vi "Autonomous Independent.vi"() -> ()   [LabVIEW 2011]
doc: "This VI is called when autonomous begins, and will automatically be terminated when autonomous ends. You can carry out timed or sensor driven robot movement independently without needing to return to the caller."
uses:
  <vilib>/Rock Robotics/WPI/Relay/WPI_RelayValue.ctl
  Robot Global Data.vi
  cupStateGlobal.vi
  <vilib>/Rock Robotics/WPI/RobotDrive/WPI_RobotDriveArcadeDrive_Standard(NoSaturation).vi
panel:
  out "Fixed Distance[m]":dbl
  in  "MotorPower 3":dbl
  in  "Slide 3":dbl(slide) scale=400.0..2000.0
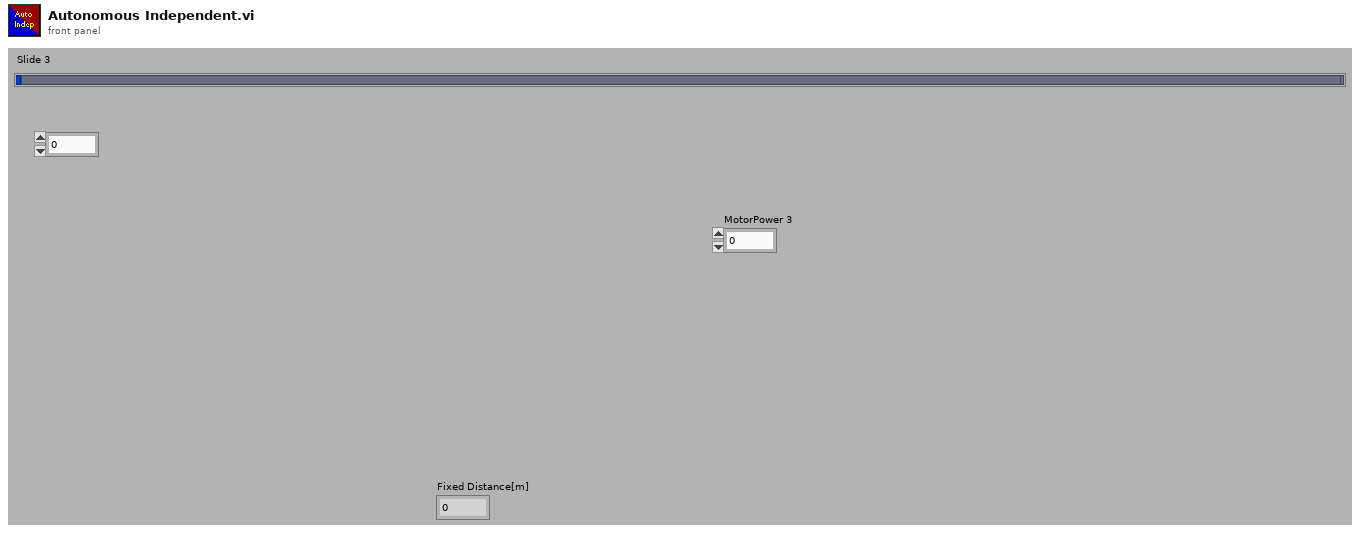
[diagram p1: front panel]
types:
  T1 = typedef "WPI_JoystickDevRef.ctl" = cluster{"Device":T2}
  T2 = typedef "WPI_JoystickDeviceEnum.ctl" = enum16{"USB 1", "USB 2", "USB 3", "USB 4", "Kinect 1", "Kinect 2"}
  T3 = typedef "WPI_DigitalInputDevRef.ctl" = cluster{"DevStatus":errorcluster, "DIO Channel":T4, "Digital Module":T5}
  T4 = typedef "FPGA_DIOChannel.ctl" = enum8{"DIO 1", "DIO 2", "DIO 3", "DIO 4", "DIO 5", "DIO 6", "DIO 7", "DIO 8", "DIO 9", "DIO 10", "DIO 11", "DIO 12", "DIO 13", "DIO 14", "Invalid"}
  T5 = typedef "FPGA_TypedefDigitalModule.ctl" = enum16{"Digital Module 1", "Digital Module 2"}
  T6 = typedef "WPI_RelayValue.ctl" = enum16{"Off", "On", "Forward", "Reverse"}
  T7 = typedef "WPI_RobotDriveDevRef.ctl" = cluster{"DevStatus":errorcluster, "Motors[]":T8[], "Square Inputs":bool, "Max Output":dbl, "Isochronous":bool}
  T8 = typedef "WPI_MotorControlDeviceRef.ctl" = cluster{"DeviceStatus":errorcluster, "Type":enum16{"PWM", "CAN"}, "PWM":cluster{"Digital Module":T5, "PWM Channel":T9, "DeadBand":T10}, "CAN":cluster{"Device Number":u8, "Control Mode":T11, "Semaphore":T12, "Max Vout":dbl}, "Invert":bool, "TransformRef":T13, "InvTransformRef":T13}
  T9 = typedef "FPGA_DIOPWMChannel.ctl" = enum8{"PWM 1", "PWM 2", "PWM 3", "PWM 4", "PWM 5", "PWM 6", "PWM 7", "PWM 8", "PWM 9", "PWM 10", "Invalid"}
  T10 = typedef "WPI_PWMDeadband.ctl" = cluster{"Name":string, "maxPositivePwm":i32, "minPositivePwm":i32, "centerPwm":i32, "maxNegativePwm":i32, "minNegativePwm":i32, "angularRange":u16}
  T11 = typedef "WPI_CANJaguar_ControlMode.ctl" = enum8{"Percent VBus", "Current", "Speed", "Position", "Voltage"}
  T12 = typedef "Semaphore RefNum" = refnum<k1>
  T13 = typedef "WPI_PWMTransform_ConPane.ctl" = refnum<vi>
  T14 = typedef "WPI_EncoderDevRef.ctl" = cluster{"DevStatus":errorcluster, "EncoderIndex":T15, "CounterIndex":T16, "DistancePerCount":dbl, "Decoding Type":T17}
  T15 = typedef "FPGA_EncoderIdx.ctl" = enum8{"Enc 0", "Enc 1", "Enc 2", "Enc 3", "Invalid"}
  T16 = typedef "FPGA_CounterCtrSystemIndex.ctl" = enum8{"Ctr 0", "Ctr 1", "Ctr 2", "Ctr 3", "Ctr 4", "Ctr 5", "Ctr 6", "Ctr 7", "Invalid"}
  T17 = typedef "WPI_EncoderType.ctl" = enum16{"1x", "2x", "4x"}
  T18 = typedef "WPI_AnalogChannelDevRef.ctl" = cluster{"DevStatus":errorcluster, "Analog Module":T19, "Analog Channel":T20}
  T19 = typedef "FPGA_TypedefAnalogModule.ctl" = enum16{"Analog Module 1", "Analog Module 2"}
  T20 = typedef "FPGA_AIChannel.ctl" = enum8{"AI 1", "AI 2", "AI 3", "AI 4", "AI 5", "AI 6", "AI 7", "AI 8", "Invalid"}
  T21 = cluster{"RightAxis":dbl, "LeftAxis":dbl, "RightHead":bool, "Left Head":bool, "Left Leg Out":bool, "Left Leg Forward":bool, "Left Leg Back":bool, "Right Leg Out":bool, "Right Leg Forward":bool, "Right Leg Back":bool}
  T22 = typedef "WPI_RelayDevRef.ctl" = cluster{"DevStatus":errorcluster, "Relay Channel":T23, "Digital Module":T5, "Relay Direction":T24}
  T23 = typedef "FPGA_DIORelayChannel.ctl" = enum8{"Relay 1", "Relay 2", "Relay 3", "Relay 4", "Relay 5", "Relay 6", "Relay 7", "Relay 8", "Invalid"}
  T24 = typedef "WPI_RelayDirection.ctl" = enum16{"Both directions", "Forward only", "Reverse only"}
  T25 = typedef "WPI_ServoDeviceRef.ctl" = cluster{"DeviceStatus":errorcluster, "Digital Module":T5, "PWM Channel":T9, "DeadBand":T10}
  T26 = cluster{"Position":cluster{"X":dbl, "Y":dbl}, "Distance (m)":dbl, "Target Found?":bool}
  T27 = cluster{"axis 1 (x)":dbl, "axis 2 (y)":dbl, "axis 3 (throttle)":dbl, "axis 4":dbl, "axis 5":dbl, "axis 6":dbl}
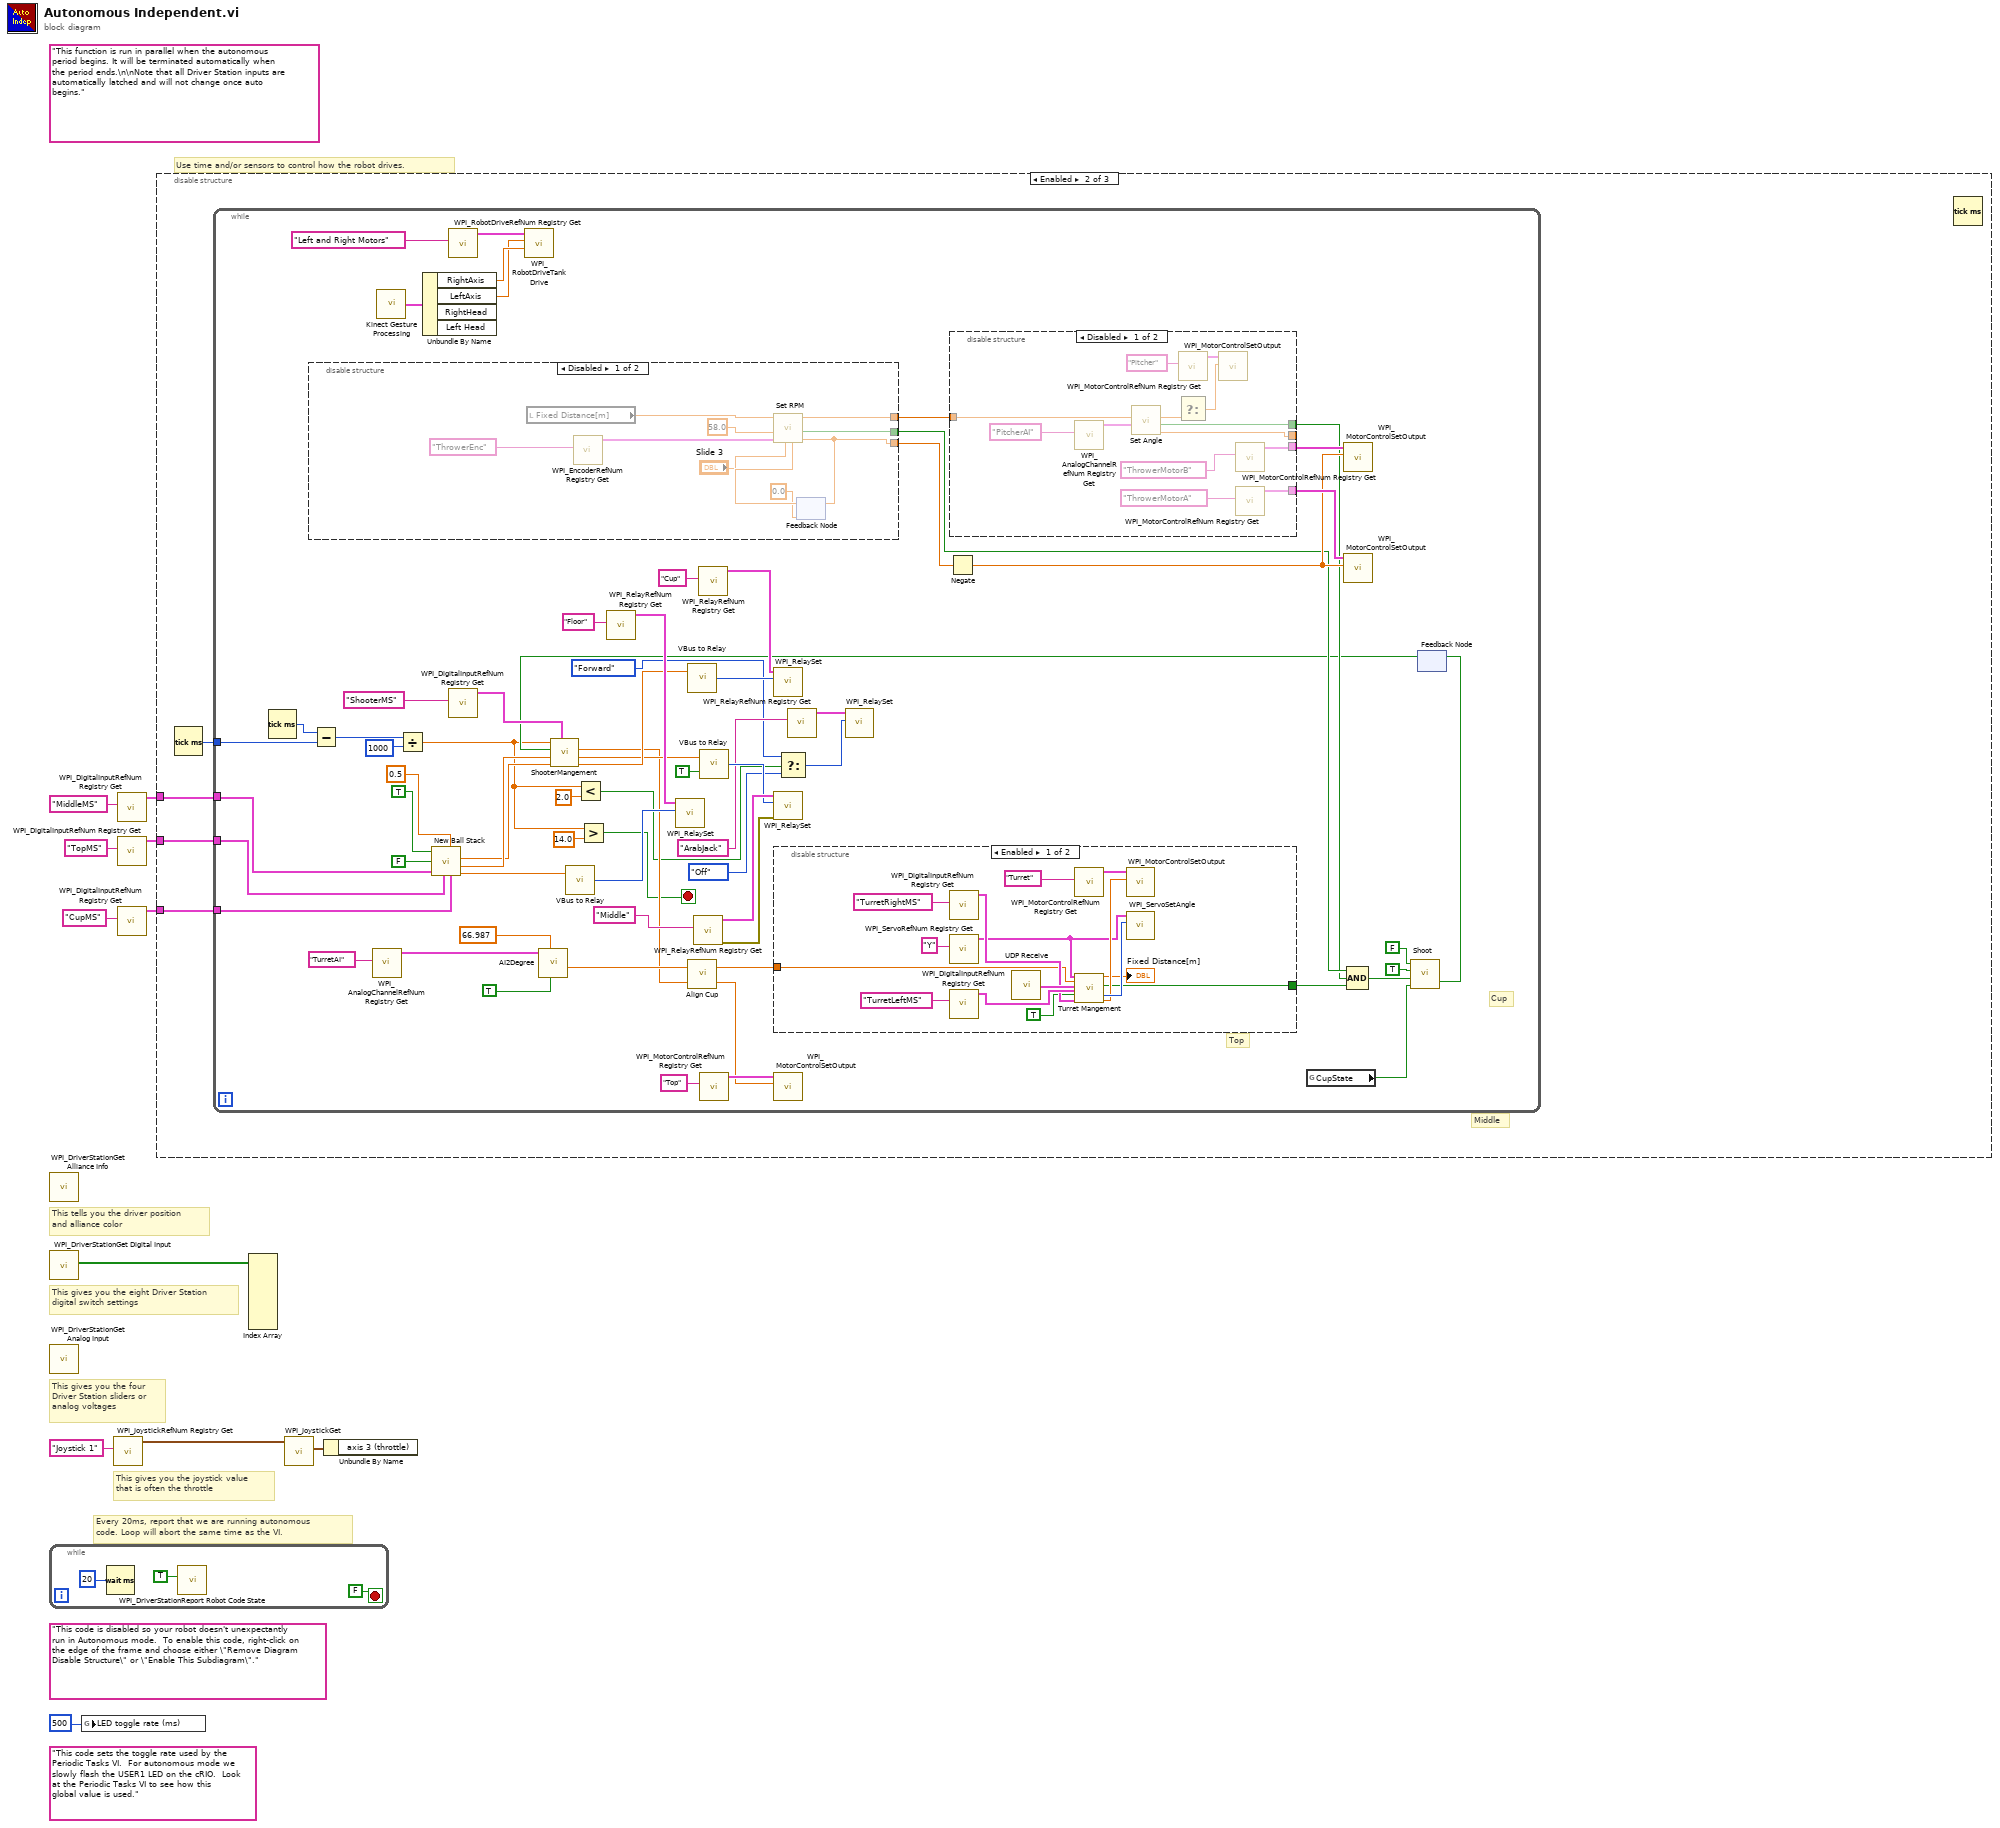
[diagram p0: block diagram]
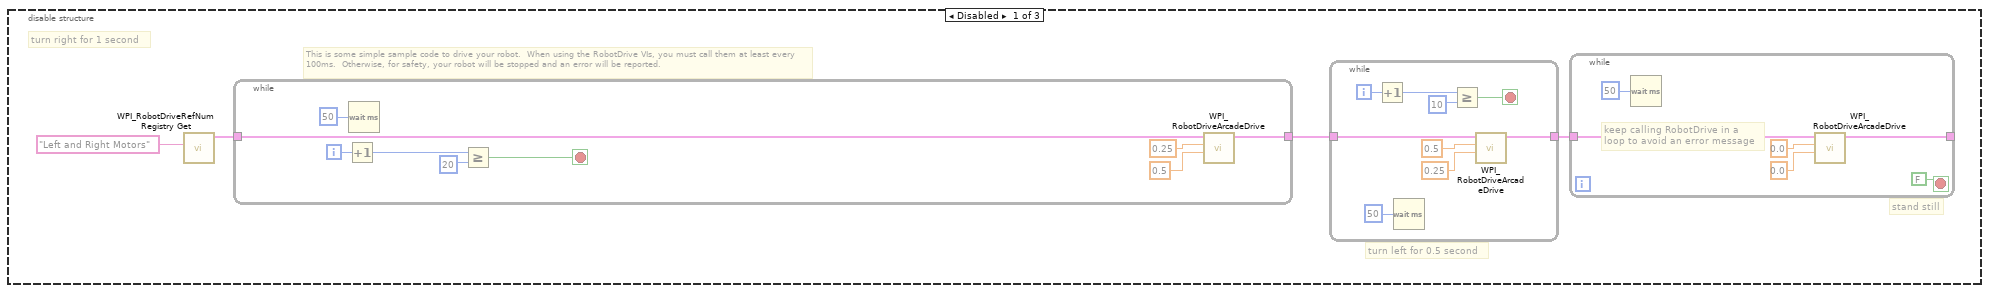
[diagram p2: hidden frame]
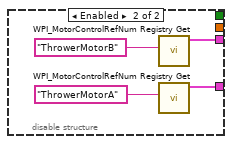
[diagram p4: hidden frame]
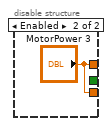
[diagram p5: hidden frame]
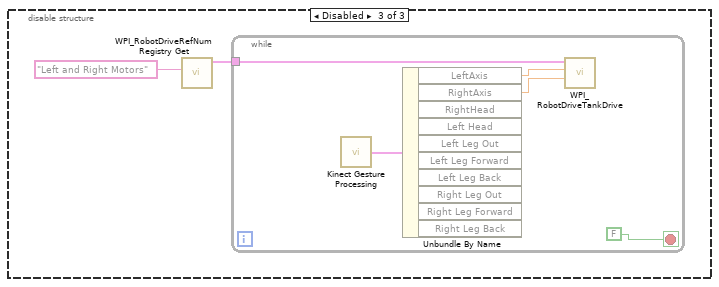
[diagram p6: hidden frame]
diagram:
  (unwired) "This code sets the toggle rate used by the Periodic Tasks VI.  For autonomous mode we slowly flash the USER1 LED on the cRIO.  Look at the Periodic Tasks VI to see how this global value is used."
  (unwired) "This code is disabled so your robot doesn't unexpectantly run in Autonomous mode.  To enable this code, right-click on the edge of the frame and choose either \"Remove Diagram Disable Structure\" or \"Enable This Subdiagram\"."
  (unwired) "This function is run in parallel when the autonomous period begins. It will be terminated automatically when the period ends.\n\nNote that all Driver Station inputs are automatically latched and will not change once auto begins."
  # "Every 20ms, report that we are running autonomous\ncode. Loop will abort the same time as the VI."
  # "This gives you the joystick value\nthat is often the throttle"
  # "Use time and/or sensors to control how the robot drives."
  # "This tells you the driver position\nand alliance color"
  # "This gives you the eight Driver Station\ndigital switch settings"
  # "This gives you the four\nDriver Station sliders or\nanalog voltages"
  n1 = call <vilib>:"WPI_DriverStationGet Alliance Info.vi"() -> ()  [unwired: 12 out]
  n2 = call <vilib>:"WPI_DriverStationGet Digital Input.vi"() -> ("Driver Station Digital Input (1-8)"=w11:bool[])  [unwired: 11 out]
  n3 = call <vilib>:"WPI_DriverStationGet Analog Input.vi"() -> ()  [unwired: 12 out]
  n4 = while {
    stop <- FALSE stop-if-true
    n5 = Wait (ms)(milliseconds to wait=u32 20) -> ()  [unwired: 1 out]
    n6 = call <vilib>:"WPI_DriverStationReport Robot Code State.vi"("Autonomous"=TRUE) -> ()  [unwired: 10 in, 1 out]
  }
  n7 = global write "Robot Global Data.vi" "LED toggle rate (ms)"(u32 500 ("LED ms toggle rate")) -> ()
  n8 = call <vilib>:"WPI_JoystickRefNum Registry Get.vi"("refnum name"="Joystick 1") -> ("JoystickDevRef"=w8:T1)  [unwired: 1 in, 9 out]
  n9 = call <vilib>:"WPI_DigitalInputRefNum Registry Get.vi"("refnum name"="MiddleMS") -> ("DigitalInputDevRef"=w1:T3)  [unwired: 9 in, 1 out]
  n10 = call <vilib>:"WPI_DigitalInputRefNum Registry Get.vi"("refnum name"="TopMS") -> ("DigitalInputDevRef"=w2:T3)  [unwired: 9 in, 1 out]
  n11 = call <vilib>:"WPI_DigitalInputRefNum Registry Get.vi"("refnum name"="CupMS") -> ("DigitalInputDevRef"=w3:T3)  [unwired: 9 in, 1 out]
  n12 = disable-structure shown="Enabled" {
    disable-tunnel: w3 -> [_ w45 _]
    disable-tunnel: w2 -> [_ w46 _]
    disable-tunnel: w1 -> [_ w44 _]
    frame Disabled {
      # "This is some simple sample code to drive your robot.  When using the RobotDrive VIs, you must call them at least every 100ms.  Otherwise, for safety, your robot will be stopped and an error will be reported."
      # "stand still"
      # "turn left for 0.5 second"
      # "turn right for 1 second"
      n13 = call <vilib>:"WPI_RobotDriveRefNum Registry Get.vi"("refnum name"="Left and Right Motors") -> ("RobotDriveDevRef"=w17:T7)  [unwired: 1 in, 9 out]
      n14 = while {
        tunnel: w17 -> [w42]
        tunnel: [w35] -> w16
        i -> [w38]
        stop <- w36 stop-if-true
        n15 = Increment(x=w38) -> (x+1=w34:i32)
        n16 = Wait (ms)(milliseconds to wait=u32 50) -> ()  [unwired: 1 out]
        n17 = Greater Or Equal?(x=w34, y=20) -> (x >= y?=w36:bool)
        n18 = call-poly <vilib>:"WPI_RobotDriveArcadeDrive.vi"("Y axis value"=0.5 ("X axis value"), "X axis value"=0.25, "RobotDriveDevRef"=w42) -> ("RobotDriveDevRef"=w35:T7)  [unwired: 1 in, 7 out]
      }
      n19 = while {
        tunnel: w16 -> [w33]
        tunnel: [w26] -> w15
        i -> [w29]
        stop <- w27 stop-if-true
        n20 = Increment(x=w29) -> (x+1=w25:i32)
        n21 = Wait (ms)(milliseconds to wait=u32 50) -> ()  [unwired: 1 out]
        n22 = Greater Or Equal?(x=w25, y=10) -> (x >= y?=w27:bool)
        n23 = call-poly <vilib>:"WPI_RobotDriveArcadeDrive.vi"("Y axis value"=0.25 ("X axis value"), "X axis value"=0.5, "RobotDriveDevRef"=w33) -> ("RobotDriveDevRef"=w26:T7)  [unwired: 1 in, 7 out]
      }
      n24 = while {
        tunnel: w15 -> [w24]
        tunnel: [w20] -> _
        stop <- FALSE stop-if-true
        # "keep calling RobotDrive in a loop to avoid an error message"
        n25 = Wait (ms)(milliseconds to wait=u32 50) -> ()  [unwired: 1 out]
        n26 = call-poly <vilib>:"WPI_RobotDriveArcadeDrive.vi"("Y axis value"=0.0 ("X axis value"), "X axis value"=0.0, "RobotDriveDevRef"=w24) -> ("RobotDriveDevRef"=w20:T7)  [unwired: 1 in, 7 out]
      }
    }
    frame Enabled {
      # "Middle"
      n27 = Tick Count (ms)() -> (millisecond timer value=w43:u32)
      n28 = while {
        tunnel: w46 -> [w102]
        tunnel: w45 -> [w101]
        tunnel: w44 -> [w100]
        tunnel: w43 -> [w63]
        stop <- w60 stop-if-true
        # "Top"
        # "Cup"
        n29 = Tick Count (ms)() -> (millisecond timer value=w62:u32)
        n30 = disable-structure shown="Disabled" {
          disable-tunnel: [w155 _] -> w74
          disable-tunnel: [w150 "MotorPower 3"] -> w109
          disable-tunnel: [w149 "MotorPower 3"] -> w106
          frame Disabled {
            n31 = local read "Fixed Distance[m]"() -> (w146:dbl)
            n32 = call <vilib>:"WPI_EncoderRefNum Registry Get.vi"("refnum name"="ThrowerEnc") -> ("EncoderDevRef"=w154:T14)  [unwired: 9 in, 1 out]
            n33 = feedback #1(0.0 ("Thrower Voltage")) -> (w152:dbl)
            n34 = call "Set RPM.vi"("Last Thrower Voltage (node)"=w152, "Position"="Slide 3", "EncoderDevRef"=w154, "Angle"=58.0, "horizontal distance to basket"=w146) -> ("Thrower Voltage"=w149:dbl, "RPM SET"=w155:bool, "angle"=w150:dbl)  [unwired: 4 in]
            n35 = feedback-in #1(w149) -> ()
          }
          frame Enabled {
          }
        }
        n36 = Subtract(x=w62, y=w63) -> (x-y=w64:u32)
        n37 = call <vilib>:"WPI_AnalogChannelRefNum Registry Get.vi"("refnum name"="TurretAI") -> ("AIDeviceRef"=w84:T18)  [unwired: 9 in, 1 out]
        n38 = call "Kinect Gesture Processing.vi"() -> ("Joystick Data"=w51:T21)  [unwired: 1 in]
        n39 = Divide(x=w64, y=u32 1000 ("milliseconds to wait")) -> (x/y=w57:dbl)
        n40 = Unbundle By Name(w51) -> ("RightAxis"=w50:dbl, "LeftAxis"=w49:dbl)  [unwired: 2 out]
        n41 = call "New Ball Stack.vi"("Suck?"=TRUE, "spinOut?"=FALSE, "MiddleMS"=w100, "TopMS"=w102, "Top Stack Speed"=0.5, "CupMS"=w101) -> ("Top"=w98:dbl, "Middle"=w99:dbl, "Floor"=w77:dbl)  [unwired: 2 in]
        n42 = call <vilib>:"WPI_RobotDriveRefNum Registry Get.vi"("refnum name"="Left and Right Motors") -> ("RobotDriveDevRef"=w48:T7)  [unwired: 9 in, 1 out]
        n43 = call <vilib>:"WPI_DigitalInputRefNum Registry Get.vi"("refnum name"="ShooterMS") -> ("DigitalInputDevRef"=w96:T3)  [unwired: 9 in, 1 out]
        n44 = call <vilib>:"WPI_RobotDriveTankDrive.vi"("Right axis value"=w50, "Left axis value"=w49, "RobotDriveDevRef"=w48) -> ()  [unwired: 7 in, 2 out]
        n45 = call "AI2Degree.vi"("Invert"=TRUE, "Calibrate"=66.987 ("y"), "AIDeviceRef"=w84) -> ("Degree"=w82:dbl)  [unwired: 8 in]
        n46 = call "VBus to Relay.vi"("Motor VBus"=w77) -> ("RelayValue"=w81:T6)  [unwired: 1 in]
        n47 = Less?(x=w57, y=2.0) -> (x < y?=w55:bool)
        n48 = Greater?(x=w57, y=14.0) -> (0:w60:bool)
        n49 = call <vilib>:"WPI_RelayRefNum Registry Get.vi"("refnum name"="Floor") -> ("RelayDevRef"=w110:T22)  [unwired: 9 in, 1 out]
        n50 = call <vilib>:"WPI_RelaySet.vi"("RelayValue"=w81, "RelayDevRef"=w110) -> ()  [unwired: 8 in, 2 out]
        n51 = call <vilib>:"WPI_RelayRefNum Registry Get.vi"("refnum name"="Middle") -> ("error out"=w91:errorcluster, "RelayDevRef"=w92:T22)  [unwired: 9 in]
        n52 = call <vilib>:"WPI_RelayRefNum Registry Get.vi"("refnum name"="Cup") -> ("RelayDevRef"=w112:T22)  [unwired: 9 in, 1 out]
        n53 = call <vilib>:"WPI_MotorControlRefNum Registry Get.vi"("refnum name"="Top") -> ("MotorControlDevRef"=w87:T8)  [unwired: 9 in, 1 out]
        n54 = Select(t=WPI_RelayValue."Forward" ("RelayValue"), s=w55, f=WPI_RelayValue."Off" ("RelayValue")) -> (s? t:f=w52:T6)
        n55 = call <vilib>:"WPI_RelayRefNum Registry Get.vi"("refnum name"="ArabJack") -> ("RelayDevRef"=w59:T22)  [unwired: 9 in, 1 out]
        n56 = call <vilib>:"WPI_RelaySet.vi"("RelayValue"=w52, "RelayDevRef"=w59) -> ()  [unwired: 8 in, 2 out]
        n57 = Negate(x=w106) -> (-x=w75:dbl)
        n58 = disable-structure shown="Disabled" {
          disable-tunnel: [w141 _] -> w73
          disable-tunnel: w109 -> [w129 _]
          disable-tunnel: [w138 w143] -> w108
          disable-tunnel: [w137 w142] -> w107
          disable-tunnel: [w132 _] -> _
          frame Disabled {
            n59 = call <vilib>:"WPI_AnalogChannelRefNum Registry Get.vi"("refnum name"="PitcherAI") -> ("AIDeviceRef"=w134:T18)  [unwired: 9 in, 1 out]
            n60 = call "Set Angle.vi"("AIDeviceRef"=w134, "Angle"=w129) -> ("Current Angle(above Horizon)"=w132:dbl, "Angle SET"=w141:bool, "Angle Motor"=w130:dbl)  [unwired: 7 in]
            n61 = call <vilib>:"WPI_MotorControlRefNum Registry Get.vi"("refnum name"="Pitcher") -> ("MotorControlDevRef"=w133:T8)  [unwired: 9 in, 1 out]
            n62 = Select(f=w130) -> (s? t:f=w131:dbl)  [unwired: 2 in]
            n63 = call <vilib>:"WPI_MotorControlSetOutput.vi"("Output"=w131, "MotorControlDevRef"=w133) -> ()  [unwired: 8 in, 2 out]
            n64 = call <vilib>:"WPI_MotorControlRefNum Registry Get.vi"("refnum name"="ThrowerMotorB") -> ("MotorControlDevRef"=w137:T8)  [unwired: 9 in, 1 out]
            n65 = call <vilib>:"WPI_MotorControlRefNum Registry Get.vi"("refnum name"="ThrowerMotorA") -> ("MotorControlDevRef"=w138:T8)  [unwired: 9 in, 1 out]
          }
          frame Enabled {
            n66 = call <vilib>:"WPI_MotorControlRefNum Registry Get.vi"("refnum name"="ThrowerMotorB") -> ("MotorControlDevRef"=w142:T8)  [unwired: 9 in, 1 out]
            n67 = call <vilib>:"WPI_MotorControlRefNum Registry Get.vi"("refnum name"="ThrowerMotorA") -> ("MotorControlDevRef"=w143:T8)  [unwired: 9 in, 1 out]
          }
        }
        n68 = global read "cupStateGlobal.vi" "CupState"() -> (w68:bool)
        n69 = call <vilib>:"WPI_MotorControlSetOutput.vi"("Output"=w75, "MotorControlDevRef"=w107) -> ()  [unwired: 8 in, 2 out]
        n70 = call <vilib>:"WPI_MotorControlSetOutput.vi"("Output"=w75, "MotorControlDevRef"=w108) -> ()  [unwired: 8 in, 2 out]
        n71 = feedback #2() -> (w66:bool)  [unwired: 1 in]
        n72 = call "ShooterMangement.vi"("Shooter MS"=w96, "Top"=w98, "Middle"=w99, "Le Shoot"=w66, "TeleOp Elapsed Seconds"=w57) -> ("Cup Gain"=w95:dbl, "Middle"=w88:dbl, "Top"=w78:dbl)  [unwired: 4 in]
        n73 = call "VBus to Relay.vi"("Motor VBus"=w95) -> ("RelayValue"=w94:T6)  [unwired: 1 in]
        n74 = call "Align Cup.vi"("Top Input"=w78, "Turret Angle"=w82) -> ("Top Output"=w80:dbl, "Turret Output"=w76:dbl)
        n75 = call "VBus to Relay.vi"("Invert Relay? (F)"=TRUE, "Motor VBus"=w88) -> ("RelayValue"=w89:T6)
        n76 = call <vilib>:"WPI_RelaySet.vi"("RelayValue"=w94, "RelayDevRef"=w112) -> ()  [unwired: 8 in, 2 out]
        n77 = call <vilib>:"WPI_RelaySet.vi"("error in (no error)"=w91, "RelayValue"=w89, "RelayDevRef"=w92) -> ()  [unwired: 7 in, 2 out]
        n78 = disable-structure shown="Enabled" {
          disable-tunnel: w76 -> [w116 _]
          disable-tunnel: [w115 _] -> w72
          frame Enabled {
            n79 = call <vilib>:"WPI_DigitalInputRefNum Registry Get.vi"("refnum name"="TurretRightMS") -> ("DigitalInputDevRef"=w120:T3)  [unwired: 9 in, 1 out]
            n80 = call <vilib>:"WPI_ServoRefNum Registry Get.vi"("refnum name"="Y") -> ("ServoDeviceRef"=w117:T25)  [unwired: 9 in, 1 out]
            n81 = call <vilib>:"WPI_DigitalInputRefNum Registry Get.vi"("refnum name"="TurretLeftMS") -> ("DigitalInputDevRef"=w121:T3)  [unwired: 9 in, 1 out]
            n82 = call "UDP Receive.vi"() -> ("Selected Target Info"=w122:T26)  [unwired: 1 in]
            n83 = call <vilib>:"WPI_MotorControlRefNum Registry Get.vi"("refnum name"="Turret") -> ("MotorControlDevRef"=w124:T8)  [unwired: 9 in, 1 out]
            n84 = call "Turret Mangement.vi"("Servo"=w117, "Straigthener"=w116, "DashBoard Info"=w122, "Left"=w121, "AutoSearch"=TRUE ("Sync cam&cannon 4"), "Right"=w120) -> ("Fixed Height[m]"=→"Fixed Distance[m]":dbl, "Locked On Target"=w115:bool, "Servo"=w123:i32, "Turret"=w119:dbl)  [unwired: 10 in]
            n85 = call <vilib>:"WPI_MotorControlSetOutput.vi"("Output"=w119, "MotorControlDevRef"=w124) -> ()  [unwired: 8 in, 2 out]
            n86 = call <vilib>:"WPI_ServoSetAngle.vi"("Angle"=w123, "ServoDeviceRef"=w117) -> ()  [unwired: 8 in, 2 out]
          }
          frame Disabled {
          }
        }
        n87 = call <vilib>:"WPI_MotorControlSetOutput.vi"("Output"=w80, "MotorControlDevRef"=w87) -> ()  [unwired: 8 in, 2 out]
        n88 = Compound Arithmetic op=AND(w74, w73, w72) -> (w71:bool)
        n89 = call "Shoot.vi"("Stack Loaded?"=w68, "Ready 2 Shoot?"=w71, "Fire"=TRUE, "Override"=FALSE) -> ("Le Fire at Will?"=w67:bool)  [unwired: 1 out]
        n90 = feedback-in #2(w67) -> ()
      }
      n91 = Tick Count (ms)() -> ()  [unwired: 1 out]
    }
    frame Disabled {
      n92 = call <vilib>:"WPI_RobotDriveRefNum Registry Get.vi"("refnum name"="Left and Right Motors") -> ("RobotDriveDevRef"=w157:T7)  [unwired: 1 in, 9 out]
      n93 = while {
        tunnel: w157 -> [w160]
        stop <- FALSE stop-if-true
        n94 = call "Kinect Gesture Processing.vi"() -> ("Joystick Data"=w163:T21)  [unwired: 1 in]
        n95 = Unbundle By Name(w163) -> ("LeftAxis"=w161:dbl, "RightAxis"=w162:dbl)  [unwired: 8 out]
        n96 = call <vilib>:"WPI_RobotDriveTankDrive.vi"("Right axis value"=w162, "Left axis value"=w161, "RobotDriveDevRef"=w160) -> ()  [unwired: 7 in, 2 out]
      }
    }
  }
  n97 = Index Array(array=w11) -> ()  [unwired: 8 in, 8 out]
  n98 = call <vilib>:"WPI_JoystickGet.vi"("JoystickDevRef"=w8) -> ("Axes"=w9:T27)  [unwired: 1 in, 5 out]
  n99 = Unbundle By Name(w9) -> ()  [unwired: 1 out]
